vi "Write PLC Data.vi"(8 "error in":errorcluster, 10 "PLC Info":T1[](array[typedef]) {"Device Reference" format="%.0x"}, 11 "File path":path=path "C:/PLCOutput.bin") -> (0 "error out":errorcluster)   [LabVIEW 2011, in "Ethernet IP Custom Device Custom Device.lvlib"]
uses:
  Ethernet IP Custom Device Custom Device.lvlib
  EIP Tag Information.ctl
  <vilib>/NI Veristand/Custom Device API/Custom Device Item Info.ctl
  <vilib>/NI Veristand/Custom Device API/Custom Device Item Ref.ctl
  L5K Data Types.ctl
  <vilib>/NI Veristand/Custom Device API/Custom Device API.lvlib
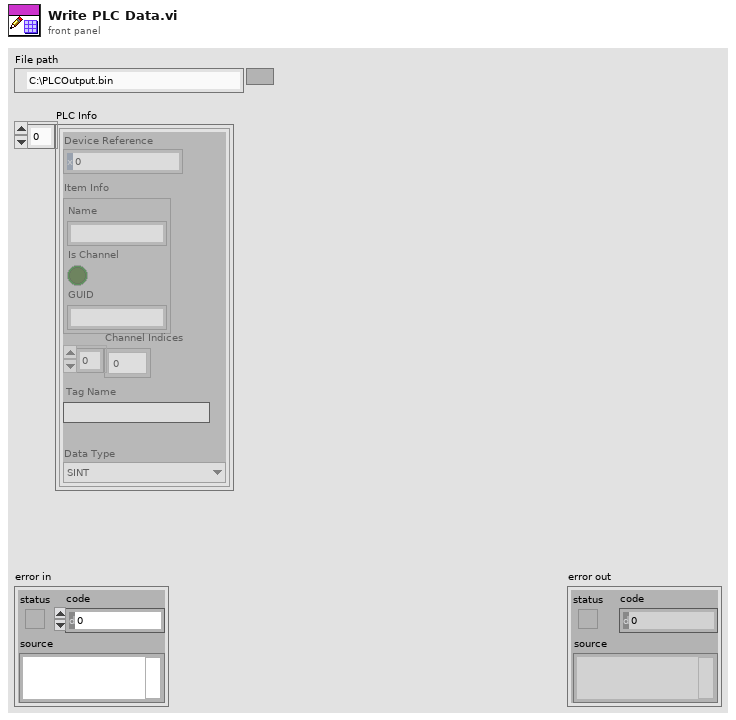
[diagram p1: front panel]
types:
  T1 = typedef "Ethernet IP Custom Device Custom Device.lvlib/EIP Tag Information.ctl" = cluster{"Item Info":T2, "Device Reference":T3, "Channel Indices":i32[], "Tag Name":string, "Data Type":T4}
  T2 = typedef "Custom Device API.lvlib/Custom Device Item Info.ctl" = cluster{"Name":string, "Is Channel":bool, "GUID":string}
  T3 = typedef "Custom Device API.lvlib/Custom Device Item Ref.ctl" = u64
  T4 = typedef "Ethernet IP Custom Device Custom Device.lvlib/L5K Data Types.ctl" = enum16{"SINT", "INT", "DINT", "REAL", "BOOL"}
  T5 = enum16{"open", "replace", "create", "open or create", "replace or create", "replace or create with confirmation"}
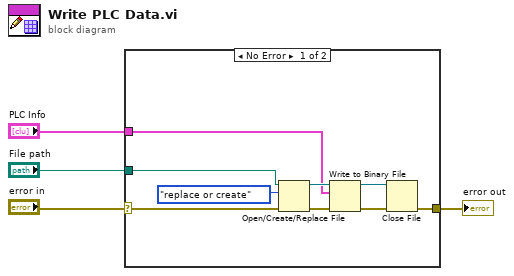
[diagram p0: block diagram]
diagram:
  n1 = case shown="No Error" "error in" {
    selector: "error in" -> [w13 w14]
    tunnel: [w12 w14] -> w3
    tunnel: "PLC Info" -> [w6 _]
    tunnel: "File path" -> [w5 _]
    frame No Error {
      n2 = Open/Create/Replace File(file path (use dialog)=w5, error in=w13, operation (0:open)=T5."replace or create") -> (refnum out=w11:refnum<file>, error out=w9:errorcluster)  [unwired: 3 in, 1 out]
      n3 = Write to Binary File(file (use dialog)=w11, data=w6, error in=w9) -> (refnum out=w10:refnum<file>, error out=w8:errorcluster)  [unwired: 3 in, 1 out]
      n4 = Close File(refnum=w10, error in=w8) -> (error out=w12:errorcluster)  [unwired: 1 out]
    }
    frame Error {
    }
  }
  "error out" <- w3
